vi "Write.vi"(8 "error in (no error)":errorcluster, 10 "dato":T1, 11 "Firebase in":refnum<class "Firebase.lvclass">) -> (0 "error out":errorcluster, 2 "Succes":bool, 3 "Firebase out":refnum<class "Firebase.lvclass">)   [LabVIEW 2019, in "Firebase.lvclass"]
uses:
  Firebase.lvclass
  <vilib>/httpClient/POSTBuffer.vi
  <vilib>/httpClient/LabVIEWHTTPClient.lvlib
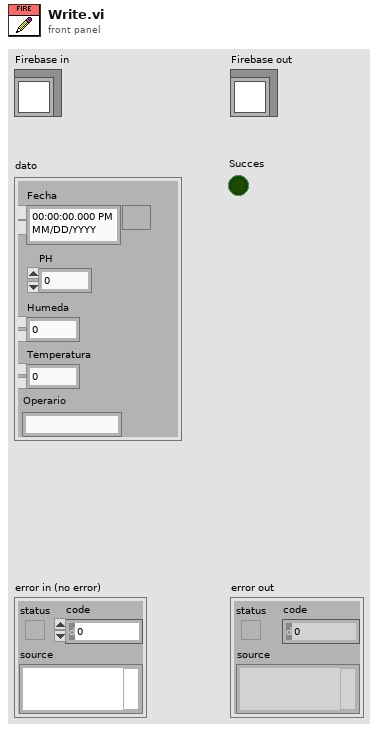
[diagram p1: front panel]
types:
  T1 = cluster{"Fecha":timestamp, "PH":dbl, "Humeda":dbl, "Temperatura":dbl, "Operario":string}
  T2 = cluster{"Dia":i32, "Hora":i32, "PH":dbl, "Humedad":dbl, "Temperatura":dbl, "Operario":string}
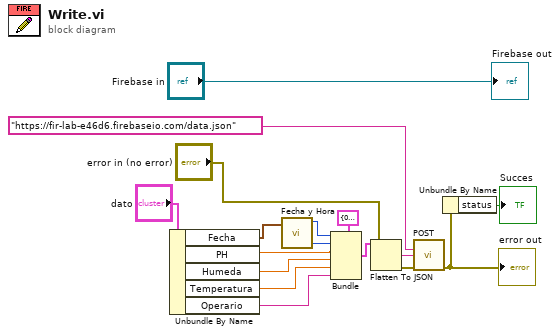
[diagram p0: block diagram]
diagram:
  n1 = Unbundle By Name("dato") -> ("Fecha"=w6:timestamp, "PH"=w11:dbl, "Humeda"=w10:dbl, "Temperatura"=w8:dbl, "Operario"=w7:string)
  n2 = call "Fecha y Hora.vi"("Fecha"=w6) -> ("Hora"=w4:i32, "Dia"=w5:i32)  [unwired: 9 in]
  n3 = Bundle(cluster=T2 {"Dia"=0, "Hora"=0, "PH"=0.0, "Humedad"=0.0, "Temperatura"=0.0, "Operario"=""} ("dato"), "Dia"=w5, "Hora"=w4, "PH"=w11, "Humedad"=w10, "Temperatura"=w8, "Operario"=w7) -> (w16:T2)
  n4 = Flatten To JSON(anything=w16, error in (no error)="error in (no error)") -> (JSON string=w15:string, 11:w14:errorcluster)  [unwired: 1 in]
  n5 = call-poly <vilib>:"POST.vi"("url"="https://fir-lab-e46d6.firebaseio.com/data.json", "buffer"=w15, "error in (no error)"=w14) -> ("error out"=w13:errorcluster)  [unwired: 9 in, 3 out]
  "error out" <- w13
  n6 = Unbundle By Name(w13) -> ("status"=→"Succes":bool)
  "Firebase out" <- "Firebase in"
